vi "FTW-JSON-Object-Join.vi"(0 "JSON Object":refnum<class "FTW-JSON.lvclass">, 5 "JSON Object to Merge":refnum<class "FTW-JSON.lvclass">, 7 "Join Mode":T1, 11 "error in":errorcluster) -> (4 "JSON Object out":refnum<class "FTW-JSON.lvclass">, 15 "error out":errorcluster)   [LabVIEW 2014, in "FTW-JSON.lvclass"]
uses:
  FTW-JSON.lvclass
  FTW-JSON-UpdateMode.ctl
  FTW-JSON.lvclass/FTW-JSON.ctl
  error/FTW-ERR-ThrowGenericError.vi
  error/FTW-ERR-ThrowError.vi
  error/FTW-ERR-NoErrorConstant.vi
  error/FTW-ERR-CallChain.vi
  string/FTW-STR-ReplaceWhitespace.vi
panel:
  # "Inputs"
  # "Outputs"
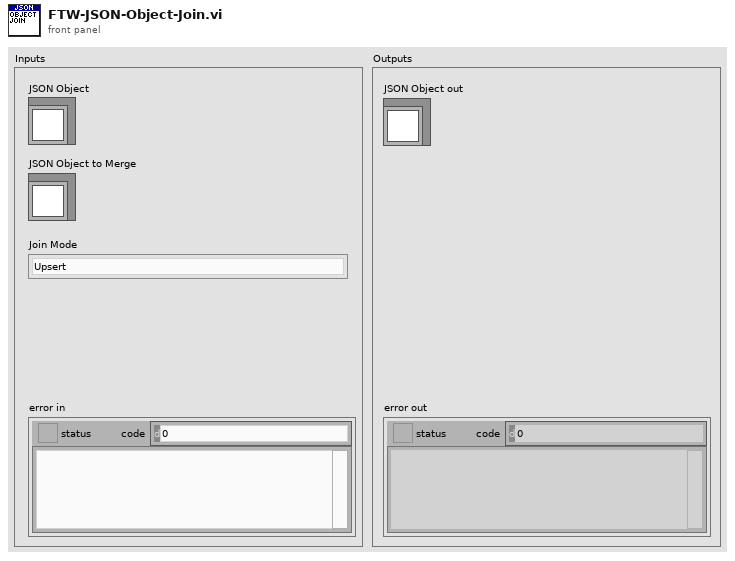
[diagram p1: front panel]
types:
  T1 = typedef "FTW-JSON.lvclass/FTW-JSON-UpdateMode.ctl" = enum16{"Upsert", "Update Only", "Insert Only"}
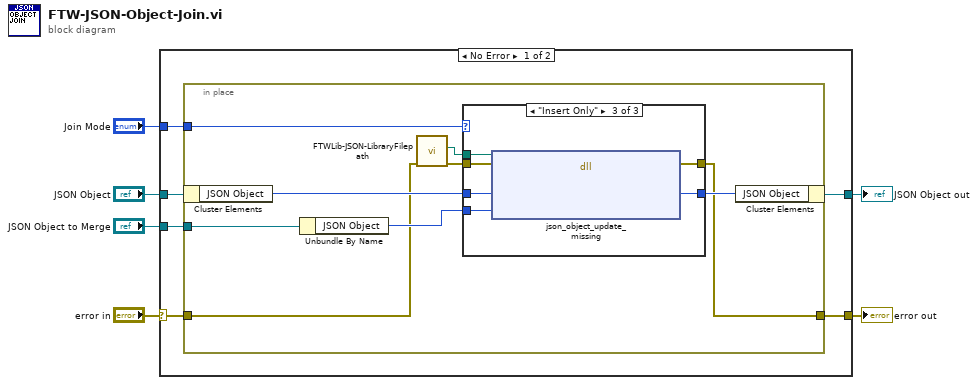
[diagram p0: block diagram]
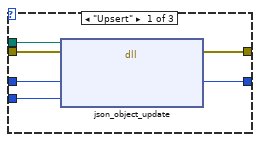
[diagram p2: hidden frame]
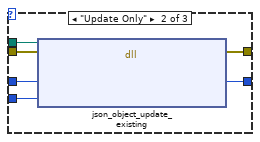
[diagram p3: hidden frame]
diagram:
  n1 = case shown="No Error" "error in" {
    selector: "error in" -> [w12 w41]
    tunnel: [w8 w41] -> w6
    tunnel: [w10 w40] -> w4
    tunnel: "JSON Object" -> [w11 w40]
    tunnel: "JSON Object to Merge" -> [w9 _]
    tunnel: "Join Mode" -> [w7 _]
    frame No Error {
      n2 = in-place {
        in-place-border: w12 -> [w13]
        in-place-border: w9 -> [w15]
        in-place-border: [w14] -> w8
        in-place-border: w7 -> [w16]
        n3 = in-place-cluster #1(w11) -> ("JSON Object"=w21:i64)
        n4 = Unbundle By Name(w15) -> ("JSON Object"=w17:i64)
        n5 = call "FTWLib-JSON-LibraryFilepath.vi"("error in"=w13) -> ("error out"=w20:errorcluster, "JSON Library Filepath"=w19:path)  [unwired: 9 in]
        n6 = case shown="\"Insert Only\"" w16 {
          tunnel: w21 -> [w27 w33 w39]
          tunnel: w20 -> [w26 w32 w38]
          tunnel: w19 -> [w25 w31 w37]
          tunnel: [w24 w30 w36] -> w18
          tunnel: [w23 w29 w35] -> w14
          tunnel: w17 -> [w22 w28 w34]
          frame "Upsert" {
            n7 = dll-call lib="?" fn="json_object_update"(path in=w25, error in=w26, "JSON Object ID"=w27, "JSON Object ID to Merge"=w22) -> (error out=w23:errorcluster, "JSON Object ID"=w24:i64)  [unwired: 3 in, 1 out]
          }
          frame "Update Only" {
            n8 = dll-call lib="?" fn="json_object_update_existing"(path in=w31, error in=w32, "JSON Object ID"=w33, "JSON Object ID to Merge"=w28) -> (error out=w29:errorcluster, "JSON Object ID"=w30:i64)  [unwired: 3 in, 1 out]
          }
          frame "Insert Only" {
            n9 = dll-call lib="?" fn="json_object_update_missing"(path in=w37, error in=w38, "JSON Object ID"=w39, "JSON Object ID to Merge"=w34) -> (error out=w35:errorcluster, "JSON Object ID"=w36:i64)  [unwired: 3 in, 1 out]
          }
        }
        n10 = in-place-cluster #1("JSON Object"=w18) -> (w10:refnum<class "FTW-JSON.lvclass">)
      }
    }
    frame Error {
    }
  }
  "error out" <- w6
  "JSON Object out" <- w4
